vi "AlliGator Baseline Simulation Check.vi"(8 "# Counts":i32, 9 "# Bins":i32, 11 "New Baseline in":dbl) -> (3 "New Baseline out":dbl)   [LabVIEW 2021, in "AlliGator Fit Method Benchmark.lvlib"]
doc: "Computes an optimized baseline."
uses:
  AlliGator Fit Method Benchmark.lvlib
panel:
  # "see the AlliGator License on the block diagram (Ctrl+E or Window:Show Block Diagram)"
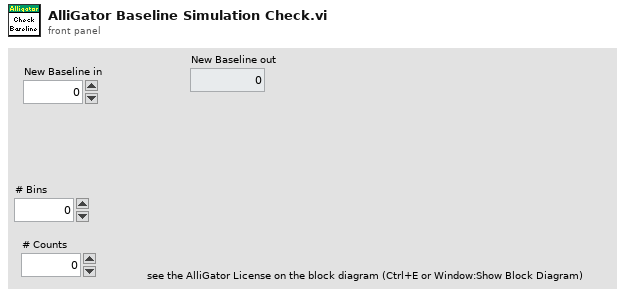
[diagram p1: front panel]
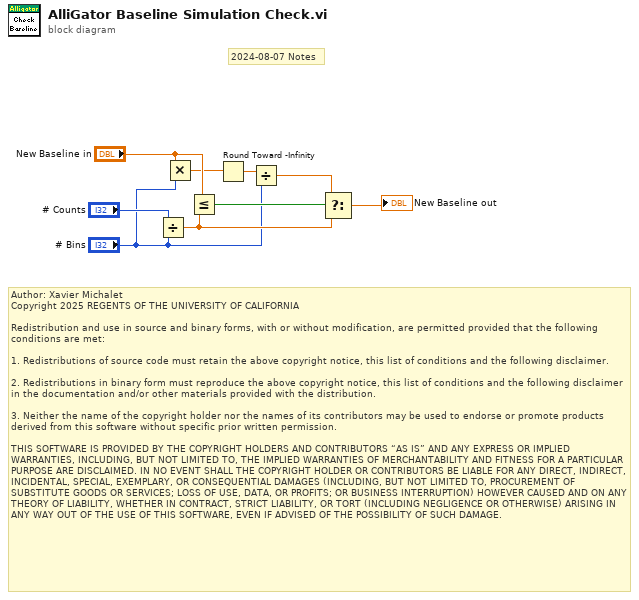
[diagram p0: block diagram]
diagram:
  # "Author: Xavier Michalet\nCopyright 2025 REGENTS OF THE UNIVERSITY OF CALIFORNIA\n\nRedistribution and use in source and binary forms, with or without modification, are permitted provided that the following conditions are met:\n\n1. Redistributions of source code must retain the above copyright notice, this list of conditions and the following disclaimer.\n\n2. Redistributions in binary form must reproduce the above copyright notice, this list of conditions and the following disclaimer in the documentation and/or other materials provided with the distribution.\n\n3. Neither the name of the copyright holder nor the names of its contributors may be used to endorse or promote products derived from this software without specific prior written permission.\n\nTHIS SOFTWARE IS PROVIDED BY THE COPYRIGHT HOLDERS AND CONTRIBUTORS “AS IS” AND ANY EXPRESS OR IMPLIED WARRANTIES, INCLUDING, BUT NOT LIMITED TO, THE IMPLIED WARRANTIES OF MERCHANTABILITY AND FITNESS FOR A PARTICULAR PURPOSE ARE DISCLAIMED. IN NO EVENT SHALL THE COPYRIGHT HOLDER OR CONTRIBUTORS BE LIABLE FOR ANY DIRECT, INDIRECT, INCIDENTAL, SPECIAL, EXEMPLARY, OR CONSEQUENTIAL DAMAGES (INCLUDING, BUT NOT LIMITED TO, PROCUREMENT OF SUBSTITUTE GOODS OR SERVICES; LOSS OF USE, DATA, OR PROFITS; OR BUSINESS INTERRUPTION) HOWEVER CAUSED AND ON ANY THEORY OF LIABILITY, WHETHER IN CONTRACT, STRICT LIABILITY, OR TORT (INCLUDING NEGLIGENCE OR OTHERWISE) ARISING IN ANY WAY OUT OF THE USE OF THIS SOFTWARE, EVEN IF ADVISED OF THE POSSIBILITY OF SUCH DAMAGE."
  # "2024-08-07 Notes"
  n1 = Divide(x="# Counts", y="# Bins") -> (x/y=w7:dbl)
  n2 = Multiply(x="New Baseline in", y="# Bins") -> (x*y=w4:dbl)
  n3 = Less Or Equal?(x="New Baseline in", y=w7) -> (x <= y?=w9:bool)
  n4 = Round Toward -Infinity(1:w4) -> (0:w3:dbl)
  n5 = Divide(x=w3, y="# Bins") -> (x/y=w1:dbl)
  n6 = Select(t=w1, s=w9, f=w7) -> (s? t:f=→"New Baseline out":dbl)
